vi "创建客户单位对象.vi"() -> (3 "引用输出":refnum<class "客户单位.lvclass">)   [LabVIEW 2013, in "个人剂量仪-云服务器.lvclass"]
panel:
  in  "企业信息":T1
  in  "用户列表":T2(array[cluster])
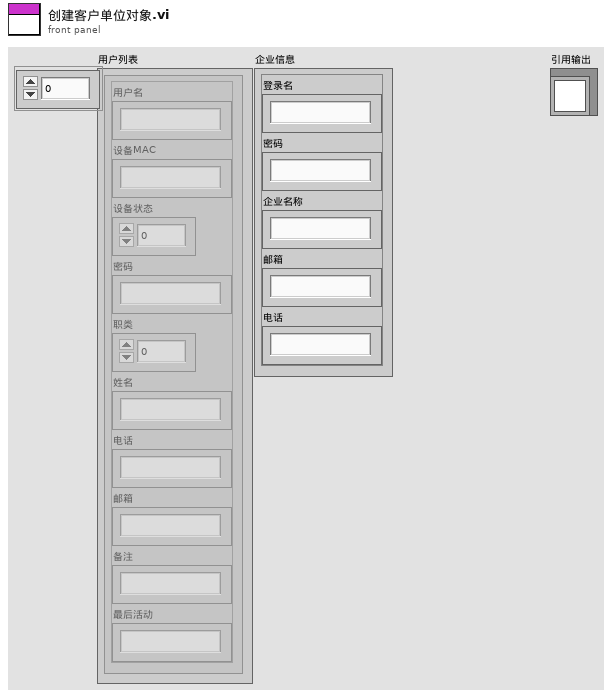
[diagram p1: front panel]
types:
  T1 = cluster{"登录名":string, "密码":string, "企业名称":string, "邮箱":string, "电话":string}
  T2 = cluster{"用户名":string, "设备MAC":string, "设备状态":i32, "密码":string, "职类":i32, "姓名":string, "电话":string, "邮箱":string, "备注":string, "最后活动":string}[]
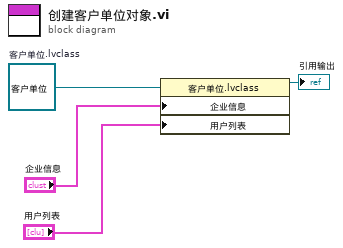
[diagram p0: block diagram]
diagram:
  w4 = refnum<class "客户单位.lvclass"> refnum  # 客户单位.lvclass
  n1 = property class="客户单位.lvclass"(reference=w4, "企业信息"="企业信息", "用户列表"="用户列表") -> (reference out=→"引用输出":refnum<class "客户单位.lvclass">)  [unwired: 1 in, 1 out]
